vi "IsEventInvalid.vi"(8 "error in (no error)":errorcluster, 11 "Event in":refnum<class "Event.lvclass">) -> (0 "error out":errorcluster, 2 "Invalid Event?":bool, 3 "Event out":refnum<class "Event.lvclass">)   [LabVIEW 2021, in "EventManagerLibrary.lvlib" / "Event.lvclass"]
uses:
  Event.lvclass
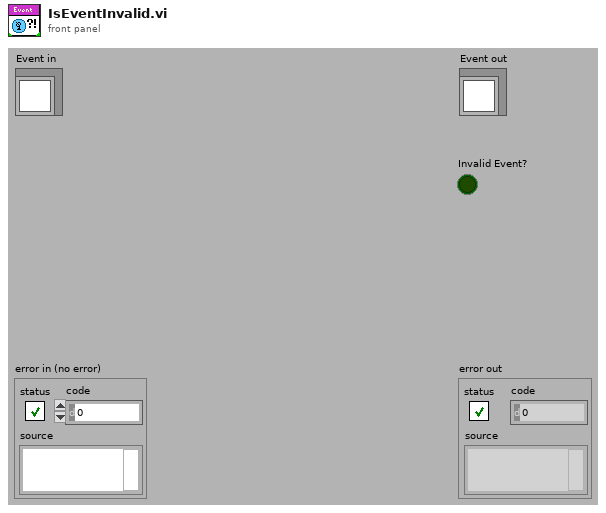
[diagram p1: front panel]
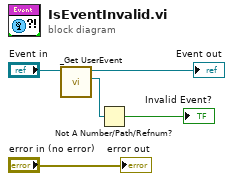
[diagram p0: block diagram]
diagram:
  n1 = call "_Get UserEvent.vi"("Event in"="Event in") -> ("UserEvent"=w1:refnum<user-event>, "Event out"=→"Event out":refnum<class "Event.lvclass">)  [unwired: 1 in, 8 out]
  n2 = Not A Number/Path/Refnum?(number/path/refnum=w1) -> (NaN/Path/Refnum?=→"Invalid Event?":bool)
  "error out" <- "error in (no error)"
